vi "HFRR ADV v04.vi"() -> ()   [LabVIEW 2025] (continued)
              n1369 = String Subset(string=w1178, offset (0)=45, length (rest)=9 ("length (rest)")) -> (substring=w1193:string)
              n1370 = Fract/Exp String To Number(string=w1193) -> (number=w1190:dbl)  [unwired: 3 in, 1 out]
              n1371 = String Subset(string=w1178, offset (0)=55, length (rest)=9 ("length (rest)")) -> (substring=w1187:string)
              n1372 = Fract/Exp String To Number(string=w1187) -> (number=w1186:dbl)  [unwired: 3 in, 1 out]
              n1373 = String Subset(string=w1178, offset (0)=25, length (rest)=9 ("length (rest)")) -> (substring=w1185:string)
              n1374 = Fract/Exp String To Number(string=w1185) -> (number=w1182:dbl)  [unwired: 3 in, 1 out]
              n1375 = String Subset(string=w1178, offset (0)=85, length (rest)=9 ("length (rest)")) -> (substring=w1179:string)
              n1376 = Fract/Exp String To Number(string=w1179) -> (number=w1177:dbl)  [unwired: 3 in, 1 out]
            }
            n1377 = Delete From Array(array=w1017, index=0) -> (array with subset deleted=w900:dbl[])  [unwired: 1 in, 1 out]
            n1378 = Delete From Array(array=w1009, index=0) -> (array with subset deleted=w898:dbl[])  [unwired: 1 in, 1 out]
            n1379 = Delete From Array(array=w1027, index=0) -> (array with subset deleted=w902:dbl[])  [unwired: 1 in, 1 out]
            n1380 = Delete From Array(array=w1007, index=0) -> (array with subset deleted=w987:dbl[])  [unwired: 1 in, 1 out]
            n1381 = Delete From Array(array=w977, index=0) -> (array with subset deleted=w904:dbl[])  [unwired: 1 in, 1 out]
            n1382 = Delete From Array(array=w1015, index=0) -> (array with subset deleted=w988:dbl[])  [unwired: 1 in, 1 out]
            n1383 = Delete From Array(array=w1025, index=0) -> (array with subset deleted=w986:dbl[])  [unwired: 1 in, 1 out]
            n1384 = Delete From Array(array=w1034, index=0) -> (array with subset deleted=w989:dbl[])  [unwired: 1 in, 1 out]
            n1385 = Bundle "Bundle"(w898, w987) -> (w1052:cluster{dbl[], dbl[]})  [unwired: 1 in]
            n1386 = Bundle "Bundle"(w902, w986) -> (w1054:cluster{dbl[], dbl[]})  [unwired: 1 in]
            n1387 = Bundle "Bundle"(w900, w988) -> (w1053:cluster{dbl[], dbl[]})  [unwired: 1 in]
            n1388 = Bundle "Bundle"(w904, w989) -> (w923:cluster{dbl[], dbl[]})  [unwired: 1 in]
            n1389 = Build Array "Build Array"(w923, w1054, w1053, w1052) -> (→"Coefficient Of Friction":cluster{dbl[], dbl[]}[])
            n1390 = Delete From Array(array=w1022, index=0) -> (array with subset deleted=w1023:dbl[])  [unwired: 1 in, 1 out]
            n1391 = Delete From Array(array=w1004, index=0) -> (array with subset deleted=w1005:dbl[])  [unwired: 1 in, 1 out]
            n1392 = Delete From Array(array=w1013, index=0) -> (array with subset deleted=w1014:dbl[])  [unwired: 1 in, 1 out]
            n1393 = Delete From Array(array=w1031, index=0) -> (array with subset deleted=w1032:dbl[])  [unwired: 1 in, 1 out]
            n1394 = Delete From Array(array=w1002, index=0) -> (array with subset deleted=w932:dbl[])  [unwired: 1 in, 1 out]
            n1395 = Delete From Array(array=w1011, index=0) -> (array with subset deleted=w933:dbl[])  [unwired: 1 in, 1 out]
            n1396 = Delete From Array(array=w1029, index=0) -> (array with subset deleted=w935:dbl[])  [unwired: 1 in, 1 out]
            n1397 = Delete From Array(array=w1020, index=0) -> (array with subset deleted=w934:dbl[])  [unwired: 1 in, 1 out]
            n1398 = Bundle "Bundle"(w898, w932) -> (w1044:cluster{dbl[], dbl[]})  [unwired: 1 in]
            n1399 = Bundle "Bundle"(w902, w934) -> (w1045:cluster{dbl[], dbl[]})  [unwired: 1 in]
            n1400 = Bundle "Bundle"(w900, w933) -> (w1043:cluster{dbl[], dbl[]})  [unwired: 1 in]
            n1401 = Bundle "Bundle"(w904, w935) -> (w922:cluster{dbl[], dbl[]})  [unwired: 1 in]
            n1402 = Delete From Array(array=w995, index=0) -> (array with subset deleted=w983:dbl[])  [unwired: 1 in, 1 out]
            n1403 = Build Array "Build Array"(w922, w1045, w1043, w1044) -> (→"Air Temperature":cluster{dbl[], dbl[]}[])
            n1404 = Delete From Array(array=w1000, index=0) -> (array with subset deleted=w985:dbl[])  [unwired: 1 in, 1 out]
            "array w/ subset deleted" <- w985
            n1405 = Delete From Array(array=w998, index=0) -> (array with subset deleted=w984:dbl[])  [unwired: 1 in, 1 out]
            n1406 = Delete From Array(array=w975, index=0) -> (array with subset deleted=w931:dbl[])  [unwired: 1 in, 1 out]
            n1407 = Bundle "Bundle"(w898, w1005) -> (w1037:cluster{dbl[], dbl[]})  [unwired: 1 in]
            n1408 = Bundle "Bundle"(w902, w1023) -> (w1036:cluster{dbl[], dbl[]})  [unwired: 1 in]
            n1409 = Bundle "Bundle"(w900, w1014) -> (w1038:cluster{dbl[], dbl[]})  [unwired: 1 in]
            n1410 = Bundle "Bundle"(w904, w1032) -> (w896:cluster{dbl[], dbl[]})  [unwired: 1 in]
            n1411 = Build Array "Build Array"(w896, w1036, w1038, w1037) -> (→"XY Graph 13":cluster{dbl[], dbl[]}[])
            n1412 = Delete From Array(array=w994, index=0) -> (array with subset deleted=w982:dbl[])  [unwired: 1 in, 1 out]
            n1413 = Delete From Array(array=w969, index=0) -> (array with subset deleted=w928:dbl[])  [unwired: 1 in, 1 out]
            n1414 = Delete From Array(array=w973, index=0) -> (array with subset deleted=w930:dbl[])  [unwired: 1 in, 1 out]
            n1415 = Delete From Array(array=w971, index=0) -> (array with subset deleted=w929:dbl[])  [unwired: 1 in, 1 out]
            n1416 = call-poly <vilib>:"Mean.vi"("X"=w987) -> ("mean"=→"КОФ4":dbl)  [unwired: 1 out]
            n1417 = call-poly <vilib>:"Mean.vi"("X"=w989) -> ("mean"=→"КОФ1":dbl)  [unwired: 1 out]
            n1418 = call-poly <vilib>:"Mean.vi"("X"=w988) -> ("mean"=→"КОФ3":dbl)  [unwired: 1 out]
            n1419 = Bundle "Bundle"(w904, w985) -> (w918:cluster{dbl[], dbl[]})  [unwired: 1 in]
            n1420 = Bundle "Bundle"(w898, w982) -> (w990:cluster{dbl[], dbl[]})  [unwired: 1 in]
            n1421 = Bundle "Bundle"(w902, w984) -> (w992:cluster{dbl[], dbl[]})  [unwired: 1 in]
            n1422 = Bundle "Bundle"(w900, w983) -> (w991:cluster{dbl[], dbl[]})  [unwired: 1 in]
            n1423 = call-poly <vilib>:"Mean.vi"("X"=w986) -> ("mean"=→"КОФ2":dbl)  [unwired: 1 out]
            n1424 = Build Array "Build Array"(w918, w992, w991, w990) -> (→"Sample Temperature":cluster{dbl[], dbl[]}[])
            n1425 = Bundle "Bundle"(w904, w931) -> (w895:cluster{dbl[], dbl[]})  [unwired: 1 in]
            n1426 = Bundle "Bundle"(w898, w928) -> (w966:cluster{dbl[], dbl[]})  [unwired: 1 in]
            n1427 = Bundle "Bundle"(w902, w930) -> (w968:cluster{dbl[], dbl[]})  [unwired: 1 in]
            n1428 = Bundle "Bundle"(w900, w929) -> (w967:cluster{dbl[], dbl[]})  [unwired: 1 in]
            n1429 = Delete From Array(array=w954, index=0) -> (array with subset deleted=w926:dbl[])  [unwired: 1 in, 1 out]
            n1430 = Delete From Array(array=w952, index=0) -> (array with subset deleted=w925:dbl[])  [unwired: 1 in, 1 out]
            n1431 = call-poly <vilib>:"Mean.vi"("X"=w984) -> ("mean"=→"CP2":dbl)  [unwired: 1 out]
            n1432 = call-poly <vilib>:"Mean.vi"("X"=w982) -> ("mean"=→"CP4":dbl)  [unwired: 1 out]
            n1433 = Build Array "Build Array"(w895, w968, w967, w966) -> (→"Humidity":cluster{dbl[], dbl[]}[])
            n1434 = call-poly <vilib>:"Mean.vi"("X"=w983) -> ("mean"=→"CP3":dbl)  [unwired: 1 out]
            n1435 = call-poly <vilib>:"Mean.vi"("X"=w985) -> ("mean"=→"CP1":dbl)  [unwired: 1 out]
            n1436 = Delete From Array(array=w956, index=0) -> (array with subset deleted=w927:dbl[])  [unwired: 1 in, 1 out]
            n1437 = Bundle "Bundle"(w935, w931) -> (w937:cluster{dbl[], dbl[]})  [unwired: 1 in]
            n1438 = Bundle "Bundle"(w932, w928) -> (w940:cluster{dbl[], dbl[]})  [unwired: 1 in]
            n1439 = Bundle "Bundle"(w934, w930) -> (w938:cluster{dbl[], dbl[]})  [unwired: 1 in]
            n1440 = Bundle "Bundle"(w933, w929) -> (w939:cluster{dbl[], dbl[]})  [unwired: 1 in]
            n1441 = Delete From Array(array=w950, index=0) -> (array with subset deleted=w924:dbl[])  [unwired: 1 in, 1 out]
            n1442 = Build Array "Build Array"(w937, w938, w939, w940) -> (→"Air Temp vs Rh":cluster{dbl[], dbl[]}[])
            n1443 = Build Array "Build Array"(w895, w918) -> (w921:cluster{dbl[], dbl[]}[])
            "XY Graph 17" <- w921
            n1444 = local write "XY Graph 16"(w921) -> ()
            n1445 = Bundle "Bundle"(w902, w926) -> (w948:cluster{dbl[], dbl[]})  [unwired: 1 in]
            n1446 = Bundle "Bundle"(w900, w925) -> (w947:cluster{dbl[], dbl[]})  [unwired: 1 in]
            n1447 = Bundle "Bundle"(w898, w924) -> (w946:cluster{dbl[], dbl[]})  [unwired: 1 in]
            n1448 = Bundle "Bundle"(w904, w927) -> (w949:cluster{dbl[], dbl[]})  [unwired: 1 in]
            n1449 = Delete From Array(array=w916, index=0) -> (array with subset deleted=w903:dbl[])  [unwired: 1 in, 1 out]
            n1450 = Delete From Array(array=w912, index=0) -> (array with subset deleted=w901:dbl[])  [unwired: 1 in, 1 out]
            n1451 = Build Array "Build Array"(w949, w948, w947, w946) -> (→"Stroke":cluster{dbl[], dbl[]}[])
            n1452 = Delete From Array(array=w910, index=0) -> (array with subset deleted=w897:dbl[])  [unwired: 1 in, 1 out]
            n1453 = Delete From Array(array=w911, index=0) -> (array with subset deleted=w899:dbl[])  [unwired: 1 in, 1 out]
            n1454 = Bundle "Bundle"(w904, w903) -> (w909:cluster{dbl[], dbl[]})  [unwired: 1 in]
            n1455 = Bundle "Bundle"(w902, w901) -> (w908:cluster{dbl[], dbl[]})  [unwired: 1 in]
            n1456 = call-poly <vilib>:"Mean.vi"("X"=w927) -> ("mean"=→"КОФ2 2":dbl)  [unwired: 1 out]
            n1457 = Bundle "Bundle"(w898, w897) -> (w906:cluster{dbl[], dbl[]})  [unwired: 1 in]
            n1458 = Bundle "Bundle"(w900, w899) -> (w907:cluster{dbl[], dbl[]})  [unwired: 1 in]
            n1459 = call-poly <vilib>:"Mean.vi"("X"=w926) -> ("mean"=→"КОФ2 3":dbl)  [unwired: 1 out]
            n1460 = call-poly <vilib>:"Mean.vi"("X"=w924) -> ("mean"=→"КОФ2 5":dbl)  [unwired: 1 out]
            n1461 = call-poly <vilib>:"Mean.vi"("X"=w925) -> ("mean"=→"КОФ2 4":dbl)  [unwired: 1 out]
            n1462 = Build Array "Build Array"(w909, w908, w907, w906) -> (→"Frequency":cluster{dbl[], dbl[]}[])
          }
          frame #2 {
          }
          frame #3 {
            n1463 = local read "String Control 4"() -> (w1220:string)
            n1464 = local read "String Control 6"() -> (w1219:string)
            n1465 = local read "String Control 8"() -> (w1218:string)
            n1466 = local read "String Control 2"() -> (w1221:string)
            n1467 = property on="OPEN" class="Bool (strict)"("Visible"=TRUE) -> ()  [unwired: 2 in, 2 out]
            n1468 = Match Pattern(string=w1219, regular expression="Frequency :- ") -> (after substring=w1244:string)  [unwired: 1 in, 3 out]
            n1469 = Match Pattern(string=w1221, regular expression="Frequency :- ") -> (after substring=w1254:string)  [unwired: 1 in, 3 out]
            n1470 = Match Pattern(string=w1220, regular expression="Frequency :- ") -> (after substring=w1249:string)  [unwired: 1 in, 3 out]
            n1471 = Match Pattern(string=w1218, regular expression="Frequency :- ") -> (after substring=w1239:string)  [unwired: 1 in, 3 out]
            n1472 = String Subset(string=w1244, length (rest)=9 ("length (rest)")) -> (substring=w1246:string)  [unwired: 1 in]
            n1473 = String Subset(string=w1254, length (rest)=9 ("length (rest)")) -> (substring=w1256:string)  [unwired: 1 in]
            n1474 = String Subset(string=w1249, length (rest)=9 ("length (rest)")) -> (substring=w1251:string)  [unwired: 1 in]
            n1475 = String Subset(string=w1239, length (rest)=9 ("length (rest)")) -> (substring=w1241:string)  [unwired: 1 in]
            n1476 = Fract/Exp String To Number(string=w1246) -> (number=w1247:dbl)  [unwired: 3 in, 1 out]
            n1477 = Fract/Exp String To Number(string=w1256) -> (number=w1257:dbl)  [unwired: 3 in, 1 out]
            n1478 = Fract/Exp String To Number(string=w1251) -> (number=w1252:dbl)  [unwired: 3 in, 1 out]
            n1479 = Fract/Exp String To Number(string=w1241) -> (number=w1242:dbl)  [unwired: 3 in, 1 out]
            n1480 = local write "freq3"(w1247) -> ()
            n1481 = local write "freq2"(w1252) -> ()
            n1482 = local write "freq1"(w1257) -> ()
            n1483 = local write "freq 4"(w1242) -> ()
            n1484 = local write "Numeric 13"(0 ("Numeric 13")) -> ()
            n1485 = local write "Numeric 11"(0 ("Numeric 11")) -> ()
            n1486 = local write "Numeric 8"(0 ("Numeric 8")) -> ()
            n1487 = local write "Numeric 12"(0 ("Numeric 12")) -> ()
            n1488 = Match Pattern(string=w1219, regular expression="Samples / cycle :- ") -> (after substring=w1227:string)  [unwired: 1 in, 3 out]
            n1489 = Match Pattern(string=w1221, regular expression="Samples / cycle :- ") -> (after substring=w1235:string)  [unwired: 1 in, 3 out]
            n1490 = Match Pattern(string=w1220, regular expression="Samples / cycle :- ") -> (after substring=w1231:string)  [unwired: 1 in, 3 out]
            n1491 = Match Pattern(string=w1218, regular expression="Samples / cycle :- ") -> (after substring=w1223:string)  [unwired: 1 in, 3 out]
            n1492 = String Subset(string=w1227, length (rest)=6 ("length (rest)")) -> (substring=w1229:string)  [unwired: 1 in]
            n1493 = String Subset(string=w1235, length (rest)=6 ("length (rest)")) -> (substring=w1237:string)  [unwired: 1 in]
            n1494 = String Subset(string=w1231, length (rest)=6 ("length (rest)")) -> (substring=w1233:string)  [unwired: 1 in]
            n1495 = String Subset(string=w1223, length (rest)=6 ("length (rest)")) -> (substring=w1225:string)  [unwired: 1 in]
            n1496 = Fract/Exp String To Number(string=w1229) -> (number=w1215:dbl)  [unwired: 3 in, 1 out]
            n1497 = Fract/Exp String To Number(string=w1237) -> (number=w1217:dbl)  [unwired: 3 in, 1 out]
            n1498 = Fract/Exp String To Number(string=w1233) -> (number=w1216:dbl)  [unwired: 3 in, 1 out]
            n1499 = Fract/Exp String To Number(string=w1225) -> (number=w1214:dbl)  [unwired: 3 in, 1 out]
            n1500 = local write "sample2"(w1216) -> ()
            n1501 = local write "sample3"(w1215) -> ()
            n1502 = local write "sample1"(w1217) -> ()
            n1503 = local write "sample4"(w1214) -> ()
          }
        }
      }
    }
    n1504 = Wait (ms)(milliseconds to wait=u32 50) -> ()  [unwired: 1 out]
    n1505 = property on="STOP 3" class="Bool (strict)"() -> ("Visible"=w828:bool)  [unwired: 2 in, 2 out]
    n1506 = case shown="True" w828 {
      frame False {
      }
      frame True {
        n1507 = case shown="True" "Save Results" {
          frame False {
          }
          frame True {
            w1738 = "\r"
            n1508 = local read "Temperature before test"() -> (w1776:dbl)
            n1509 = local read "Temperature after test"() -> (w1778:dbl)
            n1510 = local read "Humidity before test"() -> (w1775:dbl)
            n1511 = local read "Humidity after test"() -> (w1777:dbl)
            n1512 = local read "MWSD"() -> (w1779:dbl)
            n1513 = local read "WS1.4"() -> (w1782:dbl)
            n1514 = local read "AVP"() -> (w1780:dbl)
            n1515 = local read "HCF"() -> (w1781:dbl)
            n1516 = local write "Save Results"(FALSE ("OK Button 5")) -> ()
            n1517 = Number To Fractional String(number=w1778, width (-)=i16 6, precision (6)=i16 1) -> (F-format string=w1756:string)  [unwired: 1 in]
            n1518 = Number To Fractional String(number=w1779, width (-)=i16 6, precision (6)=i16 1) -> (F-format string=w1753:string)  [unwired: 1 in]
            n1519 = Number To Fractional String(number=w1780, width (-)=i16 6, precision (6)=i16 3) -> (F-format string=w1749:string)  [unwired: 1 in]
            n1520 = Number To Fractional String(number=w1777, width (-)=i16 6, precision (6)=i16 1) -> (F-format string=w1760:string)  [unwired: 1 in]
            n1521 = Number To Fractional String(number=w1781, width (-)=i16 6, precision (6)=i16 2) -> (F-format string=w1747:string)  [unwired: 1 in]
            n1522 = Number To Fractional String(number=w1782, width (-)=i16 6, precision (6)=i16 1) -> (F-format string=w1742:string)  [unwired: 1 in]
            n1523 = Number To Fractional String(number=w1776, width (-)=i16 6, precision (6)=i16 1) -> (F-format string=w1764:string)  [unwired: 1 in]
            n1524 = Number To Fractional String(number=w1775, width (-)=i16 6, precision (6)=i16 1) -> (F-format string=w1767:string)  [unwired: 1 in]
            n1525 = local read "String"() -> (w1771:string)
            n1526 = local read "FILE"() -> (w1774:string)
            n1527 = Concatenate Strings(w1771, w1774) -> (w1793:string)
            n1528 = Concatenate Strings(w1793, ".dwm" ("Substring")) -> (w1791:string)
            n1529 = Concatenate Strings(w1747, ")" ("string")) -> (w1745:string)
            n1530 = Concatenate Strings("(" ("string"), w1742, ")Microns" ("string")) -> (w1741:string)
            n1531 = Concatenate Strings("(" ("string"), w1767, " ) % RH," ("string")) -> (w1768:string)
            n1532 = Concatenate Strings("(" ("string"), w1749, ")  kPa," ("string")) -> (w1739:string)
            n1533 = String To Path(string=w1791) -> (path=w1790:path)
            n1534 = Concatenate Strings("(" ("string"), w1764, ")  Deg C ," ("string")) -> (w1763:string)
            n1535 = Concatenate Strings("(" ("string"), w1760, " ) % RH," ("string")) -> (w1759:string)
            n1536 = Concatenate Strings("(" ("string"), w1756, ")  Deg C ," ("string")) -> (w1755:string)
            n1537 = Concatenate Strings("(" ("string"), w1753, ")  Microns," ("string")) -> (w1752:string)
            n1538 = local read "REMARKS"() -> (w1773:string)
            "REMARKS 2" <- w1773
            n1539 = Concatenate Strings(w1773, w1738, " Humidity before test= " ("Substring"), w1768, w1738, " Temperature before test = " ("Substring"), w1763, w1738, " Humidity after test= " ("Substring"), w1759, w1738, "Temperature after test = " ("Substring"), w1755, w1738, "MSD = " ("Substring"), w1752, w1738, "  AVP = " ("Substring"), w1739, w1738, "  HCF                     =( " ("Substring"), w1745, w1738, " WS1.4                  = " ("Substring"), w1741, w1738) -> (w1737:string)
            "data" <- w1737
            n1540 = call <vilib>:"Write Characters To File.vi"("append to file? (new file:F)"=FALSE, "character string"=w1737, "file path (dialog if empty)"=w1790) -> ()  [unwired: 2 in, 1 out]
            n1541 = Match Pattern(string=w1737, regular expression="!") -> (after substring=→"export":string)  [unwired: 1 in, 3 out]
          }
        }
        n1542 = local read "Temperature before test"() -> (w1706:dbl)
        n1543 = local read "Humidity before test"() -> (w1708:dbl)
        n1544 = local read "Temperature after test"() -> (w1722:dbl)
        n1545 = Add(x=231.864, y=w1706) -> (x+y=w1703:dbl)
        n1546 = Add(x=231.864, y=w1722) -> (x+y=w1719:dbl)
        n1547 = local read "Humidity after test"() -> (w1724:dbl)
        n1548 = Divide(x=1705.984, y=w1703) -> (x/y=w1704:dbl)
        n1549 = Divide(x=1705.984, y=w1719) -> (x/y=w1720:dbl)
        n1550 = Subtract(x=8.017352 ("y"), y=w1704) -> (x-y=w1733:dbl)
        n1551 = expression code="10**y"(w1733) -> (w1710:dbl)
        n1552 = Subtract(x=8.017352 ("y"), y=w1720) -> (x-y=w1727:dbl)
        n1553 = expression code="10**y"(w1727) -> (w1726:dbl)
        n1554 = Multiply(x=w1708, y=w1710) -> (x*y=w1709:dbl)
        n1555 = Multiply(x=w1724, y=w1726) -> (x*y=w1725:dbl)
        n1556 = Divide(x=w1709, y=750.0) -> (x/y=w1728:dbl)
        n1557 = Divide(x=w1725, y=750.0) -> (x/y=w1729:dbl)
        n1558 = Add(x=w1728, y=w1729) -> (x+y=w1730:dbl)
        n1559 = Divide(x=w1730, y=2.0) -> (x/y=w1732:dbl)
        n1560 = local write "AVP"(w1732) -> ()
        n1561 = local read "HCF"() -> (w1715:dbl)
        n1562 = Subtract(x=1.4, y=w1732) -> (x-y=w1713:dbl)
        n1563 = local read "MWSD"() -> (w1711:dbl)
        n1564 = Multiply(x=w1713, y=w1715) -> (x*y=w1714:dbl)
        n1565 = Add(x=w1714, y=w1711) -> (x+y=→"WS1.4":dbl)
      }
    }
    n1566 = case shown="True" "Prog Uno" {
      frame False {
      }
      frame True {
        n1567 = stacked-sequence {
          frame #0 {
            n1568 = Delete(path (use dialog)=path "C:/LAB-IQ-NXT/UNOCOMPILE.bat" ("working directory")) -> ()  [unwired: 4 in, 3 out]
          }
          frame #1 {
            n1569 = local read "Com Port 1"() -> (w1306:refnum<visa-resource-name>)
            n1570 = Concatenate Strings("cmd.exe /c \"mode " ("command line"), w1306, ":1200,n,8,1\"\n" ("command line")) -> (w1311:string)
            n1571 = Concatenate Strings(w1311, "CD\\\nCD WinDucom\navrdude -C avrdude.conf -v -patmega328p -carduino -P" ("command line"), w1306, " -b115200 -D -Uflash:w:UNO_V20.hex:i\n" ("command line"), "\r") -> (w1313:string)
            "STR" <- w1313
            n1572 = call <vilib>:"Write Characters To File.vi"("append to file? (new file:F)"=FALSE, "character string"=w1313, "file path (dialog if empty)"=path "C:/LAB-IQ-NXT/UNOCOMPILE.bat" ("working directory")) -> ()  [unwired: 2 in, 1 out]
          }
          frame #2 {
            n1573 = disable-structure shown="Disabled" {
              frame Disabled {
                w1317 = "cmd.exe  /c \"C:\\LAB-IQ-NXT\\UNOCOMPILE.bat\"" ("string")
                n1574 = call <vilib>:"System Exec.vi"("expected output size  (4096)"=u32 65535, "run minimized? (F)"=FALSE, "wait until completion? (T)"=TRUE ("run minimized? (F)"), "working directory"=path "C:/LAB-IQ-NXT", "standard input"=w1317, "command line"=w1317) -> ("error out"=w1316:errorcluster, "standard output"=→"String 42":string)  [unwired: 2 in, 2 out]
                "error out 3" <- w1316
                n1575 = local write "Prog Uno"(FALSE ("run minimized? (F)")) -> ()
                n1576 = flat-sequence {
                  tunnel: w1316 -> [_]
                  frame #0 {
                  }
                }
              }
              frame Enabled {
              }
            }
          }
        }
      }
    }
    n1577 = case shown="True" "Prog Due" {
      frame False {
      }
      frame True {
        n1578 = stacked-sequence {
          frame #0 {
            n1579 = Delete(path (use dialog)=path "C:/LAB-IQ-NXT/DUECOMPILE.bat" ("working directory")) -> ()  [unwired: 4 in, 3 out]
          }
          frame #1 {
            n1580 = disable-structure shown="Disabled" {
              frame Disabled {
                n1581 = local read "visa due"() -> (w1288:string)
                n1582 = Concatenate Strings("cmd.exe /c \"mode " ("command line"), w1288, ":1200,n,8,1\"\n" ("command line")) -> (w1293:string)
                n1583 = Concatenate Strings(w1293, "CD\\\nCD WinDucom\nTIMEOUT 1\n bossac.exe -i -d --port=" ("command line"), w1288, " -U false -e -w -v -b DUE.bin -R\n" ("command line"), "\r") -> (w1295:string)
                "concatenated string 2" <- w1295
                n1584 = call <vilib>:"Write Characters To File.vi"("append to file? (new file:F)"=FALSE, "character string"=w1295, "file path (dialog if empty)"=path "C:/LAB-IQ-NXT/DUECOMPILE.bat" ("working directory")) -> ()  [unwired: 2 in, 1 out]
              }
              frame Enabled {
              }
            }
          }
          frame #2 {
            # "C:\\LAB-IQ-NXT\\DUECOMPILE.bat"
            n1585 = disable-structure shown="Disabled" {
              frame Disabled {
                w1300 = "cmd.exe  /c \"C:\\LAB-IQ-NXT\\DUECOMPILE.bat\"" ("string")
                n1586 = call <vilib>:"System Exec.vi"("expected output size  (4096)"=u32 65535, "run minimized? (F)"=FALSE, "wait until completion? (T)"=TRUE ("run minimized? (F)"), "working directory"=path "C:/LAB-IQ-NXT", "standard input"=w1300, "command line"=w1300) -> ("error out"=w1299:errorcluster, "standard output"=→"String 44":string)  [unwired: 2 in, 2 out]
                "error out 4" <- w1299
                n1587 = flat-sequence {
                  tunnel: w1299 -> [_]
                  frame #0 {
                  }
                }
              }
              frame Enabled {
              }
            }
            n1588 = local write "Prog Due"(FALSE ("Prog Due")) -> ()
          }
        }
      }
    }
    n1589 = flat-sequence {
      frame #0 {
        n1590 = local read "x = y?"() -> (w1328:bool)
        n1591 = And(x="EDIT", y=w1328) -> (x .and. y?=w1326:bool)
        n1592 = case shown="True" "SAVE" {
          frame False {
          }
          frame True {
            n1593 = stacked-sequence {
              seq-local: [w1529 _ _] -> [_ w1683 _]
              frame #0 {
                (unwired) i16 5 ("precision (6)")
                # "[CH1]    - FF\n[CH2]   - TEMPERATURE\n[CH3]    - Humidity\n[CH4]    - AIR TEMP\n[CH5]\\- Visa Uno\n[CH6] \\- Visa Due\n[CH7]  \\- file path\n[CH8]   - Displacement Gain\n[CHA]   - Stroke Gain\n[CHB]   - Stroke PID Gain\n[CHC]   -Language Selection\n[CHD]   -Power +\n[CHE]   -Power_\n[CHF]   -Heater\n[CHG]   -Humidity Wet\n[CHH]   -Humidity Dry\n[CHI]   -Integral Time"
                n1594 = local read "Com Port 1"() -> (w1520:refnum<visa-resource-name>)
                n1595 = local read "AIR TEMPERATURE :"() -> (w1516:dbl)
                n1596 = local read "DISPLACEMENT :"() -> (w1514:dbl)
                n1597 = local read "HUMIDITY:"() -> (w1515:dbl)
                n1598 = local read "Com Port 2"() -> (w1519:refnum<visa-resource-name>)
                n1599 = local read "TEMPERATURE :"() -> (w1517:dbl)
                n1600 = local read "Stroke PID Gains"() -> (w1580:T8)
                n1601 = local read "FRIC. FORCE :"() -> (w1518:dbl)
                n1602 = local read "STROKE GAIN :"() -> (w1513:dbl)
                n1603 = Unbundle By Name(w1580) -> ("Proportional Gain (Kc)"=w1579:dbl, "Integral Time (Ti, min)"=w1521:dbl)
                n1604 = local read "CH-HUMIDITY DRY"() -> (w1532:u16)
                n1605 = Path To String(path="File Path") -> (string=w1602:string)
                n1606 = local read "Language Selection"() -> (w1577:enum16{"English", "Russian"})
                n1607 = local read "CH-POWER +"() -> (w1544:u16)
                n1608 = local read "CH-HUMIDITY WET"() -> (w1535:u16)
                n1609 = Number To Fractional String(number=w1515, width (-)=i16 10 ("precision (6)"), precision (6)=i16 5) -> (F-format string=w1627:string)  [unwired: 1 in]
                n1610 = Concatenate Strings(w1602, "\\" ("string")) -> (w1601:string)
                n1611 = local read "CH-POWER -"() -> (w1541:u16)
                n1612 = Number To Fractional String(number=w1517, width (-)=i16 10 ("precision (6)"), precision (6)=i16 5) -> (F-format string=w1633:string)  [unwired: 1 in]
                n1613 = Number To Fractional String(number=w1516, width (-)=i16 10 ("precision (6)"), precision (6)=i16 5) -> (F-format string=w1621:string)  [unwired: 1 in]
                n1614 = Number To Fractional String(number=w1514, width (-)=i16 10 ("precision (6)"), precision (6)=i16 5) -> (F-format string=w1594:string)  [unwired: 1 in]
                n1615 = local read "CH-HEATER"() -> (w1538:u16)
                n1616 = Number To Fractional String(number=w1513, width (-)=i16 10 ("precision (6)"), precision (6)=i16 5) -> (F-format string=w1593:string)  [unwired: 1 in]
                n1617 = Number To Fractional String(number=w1518, width (-)=i16 10 ("precision (6)"), precision (6)=i16 5) -> (F-format string=w1634:string)  [unwired: 1 in]
                n1618 = Number To Fractional String(number=w1579, width (-)=i16 10 ("precision (6)"), precision (6)=i16 5) -> (F-format string=w1581:string)  [unwired: 1 in]
                n1619 = Number To Fractional String(number=w1577, width (-)=i16 10 ("precision (6)"), precision (6)=i16 5) -> (F-format string=w1573:string)  [unwired: 1 in]
                n1620 = Number To Fractional String(number=w1544, width (-)=i16 10 ("precision (6)"), precision (6)=i16 5) -> (F-format string=w1567:string)  [unwired: 1 in]
                n1621 = Number To Fractional String(number=w1541, width (-)=i16 10 ("precision (6)"), precision (6)=i16 5) -> (F-format string=w1564:string)  [unwired: 1 in]
                n1622 = Number To Fractional String(number=w1538, width (-)=i16 10 ("precision (6)"), precision (6)=i16 5) -> (F-format string=w1559:string)  [unwired: 1 in]
                n1623 = Number To Fractional String(number=w1535, width (-)=i16 10 ("precision (6)"), precision (6)=i16 5) -> (F-format string=w1556:string)  [unwired: 1 in]
                n1624 = Number To Fractional String(number=w1532, width (-)=i16 10 ("precision (6)"), precision (6)=i16 5) -> (F-format string=w1551:string)  [unwired: 1 in]
                n1625 = Concatenate Strings("[CH1]" ("string"), w1634, " - FF" ("string"), "\r") -> (w1632:string)
                n1626 = Concatenate Strings("[CH3]" ("string"), w1627, " - Humidity" ("string"), "\r") -> (w1624:string)
                n1627 = Concatenate Strings("[CH7]" ("string"), w1601, "- file path" ("string"), "\r") -> (w1604:string)
                n1628 = Number To Fractional String(number=w1521, width (-)=i16 10 ("precision (6)"), precision (6)=i16 5) -> (F-format string=w1525:string)  [unwired: 1 in]
                n1629 = Concatenate Strings("[CH6]" ("string"), w1519, "- Visa Due" ("string"), "\r") -> (w1605:string)
                n1630 = Concatenate Strings("[CH8]" ("string"), w1594, "- Displacement Gain" ("string"), "\r") -> (w1597:string)
                n1631 = Concatenate Strings("[CHA]" ("string"), w1593, "- Stroke Gain" ("string"), "\r") -> (w1587:string)
                n1632 = Concatenate Strings("[CH5]" ("string"), w1520, "- Visa Uno" ("string"), "\r") -> (w1610:string)
                n1633 = Concatenate Strings("[CH4]" ("string"), w1621, " - AIR TEMP" ("string"), "\r") -> (w1617:string)
                n1634 = Concatenate Strings("[CH2]" ("string"), w1633, " - TEMPERATURE" ("string"), "\r") -> (w1631:string)
                n1635 = Concatenate Strings("[CHC]" ("string"), w1573, "-Language Selection" ("string"), "\r") -> (w1570:string)
                n1636 = Concatenate Strings("[CHD]" ("string"), w1567, "-Power +" ("string"), "\r") -> (w1549:string)
                n1637 = Concatenate Strings("[CHE]" ("string"), w1564, "-Power_" ("string"), "\r") -> (w1548:string)
                n1638 = Concatenate Strings("[CHF]" ("string"), w1559, "-Heater" ("string"), "\r") -> (w1547:string)
                n1639 = Concatenate Strings("[CHB]" ("string"), w1581, "- Stroke PID Gain" ("string"), "\r") -> (w1578:string)
                n1640 = Concatenate Strings("[CHG]" ("string"), w1556, "-Humidity Wet" ("string"), "\r") -> (w1546:string)
                n1641 = Concatenate Strings("[CHH]" ("string"), w1551, "-Humidity Dry" ("string"), "\r") -> (w1545:string)
                n1642 = Concatenate Strings("[CHI]" ("string"), w1525, "-Integral Time " ("string"), "\r") -> (w1522:string)
                n1643 = Concatenate Strings(w1632, w1631, w1624, w1617, w1610, w1605, w1604, w1597, w1587, w1578, w1570, w1549, w1548, w1547, w1546, w1545, w1522) -> (w1529:string)
                "gain" <- w1529
              }
              frame #1 {
                n1644 = local read "AIR TEMP INTERCEPT:"() -> (w1646:dbl)
                n1645 = local read "TEMP INTERCEPT:"() -> (w1645:dbl)
                n1646 = local read "Com Port 3"() -> (w1655:refnum<visa-resource-name>)
                n1647 = local read "LvdtOff"() -> (w1648:dbl)
                n1648 = Number To Fractional String(number=w1645, width (-)=i16 10 ("precision (6)"), precision (6)=i16 5) -> (F-format string=w1671:string)  [unwired: 1 in]
                n1649 = Number To Fractional String(number=w1646, width (-)=i16 10 ("precision (6)"), precision (6)=i16 5) -> (F-format string=w1678:string)  [unwired: 1 in]
                n1650 = Number To Fractional String(number=w1648, width (-)=i16 10 ("precision (6)"), precision (6)=i16 5) -> (F-format string=w1652:string)  [unwired: 1 in]
                n1651 = Concatenate Strings("[CHK]" ("string"), w1671, "-TEMP INTERCEPT" ("string"), "\r") -> (w1667:string)
                n1652 = Concatenate Strings("[CHJ]" ("string"), w1678, "-AIR TEMP INTERCEPT" ("string"), "\r") -> (w1668:string)
                n1653 = Concatenate Strings("[SNO]" ("string"), "S.NO", "-" ("string"), "\r") -> (w1663:string)
                n1654 = Concatenate Strings("[CHL]" ("string"), w1655, "- Visa humid" ("string"), "\r") -> (w1658:string)
                n1655 = Concatenate Strings("[CHI]" ("string"), w1652, "-LVDT Position Offset" ("string"), "\r") -> (w1647:string)
                n1656 = Concatenate Strings(w1683, w1668, w1667, w1663, w1658, w1647) -> (w1682:string)
                n1657 = String To Path(string="C:\\LAB-IQ-NXT\\calibrate WO 2464.dcf") -> (path=w1656:path)
                n1658 = call <vilib>:"Write Characters To File.vi"("append to file? (new file:F)"=FALSE, "character string"=w1682, "file path (dialog if empty)"=w1656) -> ()  [unwired: 2 in, 1 out]
              }
              frame #2 {
                n1659 = local write "Lan flag"(0.0 ("Lan flag")) -> ()
                n1660 = local write "Re-Initialise"(TRUE ("Re-Initialise")) -> ()
                n1661 = local write "conststatus"(0.0 ("rpm value : 2")) -> ()
                n1662 = local write "SAVE"(FALSE ("OK Button 14")) -> ()
              }
            }
          }
        }
        n1663 = case shown="False" w1326 {
          tunnel: [u8 2 ("Disabled") u8 0 ("Disabled")] -> w1325
          tunnel: [w1688 TRUE ("Visible")] -> w1324
          frame False {
            w1688 = FALSE ("Visible")
            n1664 = local write "EDIT 2"(w1688) -> ()
          }
          frame True {
          }
        }
        n1665 = property on="Tab Control" class="TabCtl (strict)"("Visible"=w1324) -> ()  [unwired: 2 in, 2 out]
        n1666 = property on="EDIT 2" class="Bool (strict)"("Visible"=w1324) -> ()  [unwired: 2 in, 2 out]
        n1667 = property on="TEMPERATURE :" class="DigNum (strict)"("Disabled"=w1325) -> ()  [unwired: 2 in, 2 out]
        n1668 = property on="SAVE" class="Bool (strict)"("Visible"=w1324) -> ()  [unwired: 2 in, 2 out]
        n1669 = property on="AIR TEMPERATURE :" class="DigNum (strict)"("Disabled"=w1325) -> ()  [unwired: 2 in, 2 out]
        n1670 = property on="SPEED OUT:" class="DigNum (strict)"("Disabled"=w1325) -> ()  [unwired: 2 in, 2 out]
        n1671 = property on="HUMIDITY:" class="DigNum (strict)"("Disabled"=w1325) -> ()  [unwired: 2 in, 2 out]
        n1672 = property on="FRIC. FORCE :" class="DigNum (strict)"("Disabled"=w1325) -> ()  [unwired: 2 in, 2 out]
        n1673 = property on="Tab Control 7" class="TabCtl (strict)"("Disabled"=w1325) -> ()  [unwired: 2 in, 2 out]
        n1674 = property on="Language Selection" class="Enum (strict)"("Visible"=w1324) -> ()  [unwired: 2 in, 2 out]
        n1675 = property on="File Path" class="Path"("Disabled"=w1325) -> ()  [unwired: 2 in, 2 out]
        n1676 = property on="TEMP INTERCEPT:" class="DigNum (strict)"("Disabled"=w1325) -> ()  [unwired: 2 in, 2 out]
        n1677 = property on="visa due" class="CmbBox"("Disabled"=w1325) -> ()  [unwired: 2 in, 2 out]
        n1678 = property on="AIR TEMP INTERCEPT:" class="DigNum (strict)"("Disabled"=w1325) -> ()  [unwired: 2 in, 2 out]
        n1679 = property on="CH-HUMIDITY DRY" class="DigNum (strict)"("Disabled"=w1325) -> ()  [unwired: 2 in, 2 out]
        n1680 = property on="CH-HUMIDITY WET" class="DigNum (strict)"("Disabled"=w1325) -> ()  [unwired: 2 in, 2 out]
        n1681 = property on="CH-POWER -" class="DigNum (strict)"("Disabled"=w1325) -> ()  [unwired: 2 in, 2 out]
        n1682 = property on="CH-HEATER" class="DigNum (strict)"("Disabled"=w1325) -> ()  [unwired: 2 in, 2 out]
        n1683 = property on="CH-POWER +" class="DigNum (strict)"("Disabled"=w1325) -> ()  [unwired: 2 in, 2 out]
        n1684 = property on="SrvM CP" class="Bool (strict)"("Disabled"=w1325) -> ()  [unwired: 2 in, 2 out]
        n1685 = property on="Stroke PID Gains" class="Clust (strict)"("Disabled"=w1325) -> ()  [unwired: 2 in, 2 out]
        n1686 = property on="STROKE GAIN :" class="DigNum (strict)"("Disabled"=w1325) -> ()  [unwired: 2 in, 2 out]
        n1687 = property on="LvdtOff" class="DigNum (strict)"("Disabled"=w1325) -> ()  [unwired: 2 in, 2 out]
        n1688 = property on="DISPLACEMENT :" class="DigNum (strict)"("Disabled"=w1325) -> ()  [unwired: 2 in, 2 out]
        n1689 = property on="Port 2 Error" class="Clust (strict)"("Visible"="EDIT") -> ()  [unwired: 2 in, 2 out]
        n1690 = property on="Port 1 Error" class="Clust (strict)"("Visible"="EDIT") -> ()  [unwired: 2 in, 2 out]
        n1691 = stacked-sequence {
          frame #0 {
            n1692 = local read "EDIT"() -> (w1376:bool)
            n1693 = case shown="True" w1376 {
              tunnel: [u8 2 ("Disabled") u8 0 ("Disabled")] -> _
              frame False {
                w1378 = FALSE
                n1694 = local write "Password"("") -> ()
                n1695 = property on="ENTER THE NEW PASSWORD" class="Str"("Visible"=w1378) -> ()  [unwired: 2 in, 2 out]
                n1696 = property on="ENTER CURRENT PASSWORD" class="Str"("Visible"=w1378) -> ()  [unwired: 2 in, 2 out]
                n1697 = property on="SrvM CP" class="Bool (strict)"("Visible"=w1378) -> ()  [unwired: 2 in, 2 out]
                n1698 = property on="Password" class="Str"("Visible"=w1378) -> ()  [unwired: 2 in, 2 out]
                n1699 = local write "x = y?"(w1378) -> ()
                n1700 = local write "SrvM CP"(w1378) -> ()
                n1701 = property on="message" class="Str"("Visible"=w1378) -> ()  [unwired: 2 in, 2 out]
              }
              frame True {
                w1381 = TRUE
                n1702 = property on="SrvM CP" class="Bool (strict)"("Visible"=w1381) -> ()  [unwired: 2 in, 2 out]
                n1703 = property on="Password" class="Str"("Visible"=w1381) -> ()  [unwired: 2 in, 2 out]
              }
            }
            "dipl pwd" <- "@143$\n" ("dipl pwd")
          }
          frame #1 {
            # "Gain password"
            n1704 = String To Byte Array(string="ENTER CURRENT PASSWORD") -> (unsigned byte array=w1386:u8[])
            n1705 = Search 1D Array(1D array=w1386, element=u8 10) -> (index of element=w1389:i32)  [unwired: 1 in]
            n1706 = Index Array(array=w1386, index=w1389) -> (element=w1385:u8)
            n1707 = Equal?(x=w1385, y=10) -> (x = y?=w1383:bool)
            n1708 = case shown="True" w1383 {
              frame False {
                n1709 = property on="ENTER THE NEW PASSWORD" class="Str"("Visible"=FALSE) -> ()  [unwired: 2 in, 2 out]
              }
              frame True {
                # "password"
                # "change password logic"
                n1710 = local read "dipl pwd"() -> (w1396:string)
                n1711 = local read "ENTER CURRENT PASSWORD"() -> (w1402:string)
                n1712 = String To Byte Array(string=w1402) -> (unsigned byte array=w1404:u8[])
                n1713 = Array Size(array=w1404) -> (size(s)=w1401:i32)
                n1714 = String To Byte Array(string=w1396) -> (unsigned byte array=w1397:u8[])
                n1715 = Array Size(array=w1397) -> (size(s)=w1399:i32)
                n1716 = for {
                  N: w1401 -> [_]
                  tunnel: w1404 -> [w1428]
                  tunnel: [w1426] -> w1405 mode=indexing
                  tunnel: w1401 -> [w1420]
                  i -> [w1421]
                  n1717 = Decrement(x=w1420) -> (x-1=w1418:i32)
                  n1718 = Index Array(array=w1428, index=w1421) -> (element=w1422:u8)
                  n1719 = Equal?(x=w1421, y=w1418) -> (x = y?=w1419:bool)
                  n1720 = Number To Decimal String(number=w1422) -> (decimal integer string=w1427:string)  [unwired: 1 in]
                  n1721 = Select(t="", s=w1419, f="\r") -> (s? t:f=w1424:string)
                  n1722 = Concatenate Strings(w1427, w1424) -> (w1426:string)
                }
                n1723 = for {
                  N: w1399 -> [_]
                  tunnel: w1397 -> [w1416]
                  tunnel: [w1414] -> w1398 mode=indexing
                  tunnel: w1399 -> [w1411]
                  i -> [w1412]
                  n1724 = Decrement(x=w1411) -> (x-1=w1410:i32)
                  n1725 = Index Array(array=w1416, index=w1412) -> (element=w1415:u8)
                  n1726 = Equal?(x=w1412, y=w1410) -> (x = y?=w1409:bool)
                  n1727 = Number To Decimal String(number=w1415) -> (decimal integer string=w1413:string)  [unwired: 1 in]
                  n1728 = Select(t="", s=w1409, f="\r") -> (s? t:f=w1406:string)
                  n1729 = Concatenate Strings(w1413, w1406) -> (w1414:string)
                }
                n1730 = local read "string"() -> (w1403:string)
                n1731 = Concatenate Strings(w1405) -> (w1393:string)
                n1732 = Concatenate Strings(w1398) -> (w1392:string)
                n1733 = Concatenate Strings(w1403) -> (w1400:string)
                n1734 = Equal?(x=w1393, y=w1392) -> (x = y?=w1391:bool)
                n1735 = Equal?(x=w1393, y=w1400) -> (x = y?=w1395:bool)
                n1736 = Or(x=w1395, y=w1391) -> (x .or. y?=w1394:bool)
                n1737 = case shown="True" w1394 {
                  frame False {
                  }
                  frame True {
                    n1738 = property on="ENTER THE NEW PASSWORD" class="Str"("Visible"=TRUE) -> ()  [unwired: 2 in, 2 out]
                  }
                }
              }
            }
          }
          frame #2 {
            n1739 = String To Byte Array(string="ENTER THE NEW PASSWORD") -> (unsigned byte array=w1431:u8[])
            n1740 = Search 1D Array(1D array=w1431, element=u8 10) -> (index of element=w1435:i32)  [unwired: 1 in]
            n1741 = Index Array(array=w1431, index=w1435) -> (element=w1433:u8)
            n1742 = Equal?(x=w1433, y=10) -> (x = y?=w1430:bool)
            n1743 = case shown="True" w1430 {
              frame False {
              }
              frame True {
                n1744 = local read "ENTER THE NEW PASSWORD"() -> (w1438:string)
                n1745 = String To Byte Array(string=w1438) -> (unsigned byte array=w1443:u8[])
                n1746 = Array Size(array=w1443) -> (size(s)=w1440:i32)
                n1747 = for {
                  N: w1440 -> [_]
                  tunnel: w1443 -> [w1456]
                  tunnel: [w1453] -> w1445 mode=indexing
                  tunnel: w1440 -> [w1448]
                  i -> [w1446]
                  n1748 = Index Array(array=w1456, index=w1446) -> (element=w1455:u8)
                  n1749 = Decrement(x=w1448) -> (x-1=w1449:i32)
                  n1750 = Equal?(x=w1446, y=w1449) -> (x = y?=w1450:bool)
                  n1751 = Number To Decimal String(number=w1455) -> (decimal integer string=w1454:string)  [unwired: 1 in]
                  n1752 = Select(t="", s=w1450, f="\r") -> (s? t:f=w1447:string)
                  n1753 = Concatenate Strings(w1454, w1447) -> (w1453:string)
                }
                n1754 = local write "SrvM CP"(FALSE) -> ()
                n1755 = local write "EDIT"(FALSE) -> ()
                n1756 = local read "file path"() -> (w1437:path)
                n1757 = Concatenate Strings(w1445) -> (w1439:string)
                n1758 = Delete(path (use dialog)=w1437) -> (deleted path=w1441:path)  [unwired: 4 in, 2 out]
                n1759 = call <vilib>:"Write Characters To File.vi"("append to file? (new file:F)"=FALSE, "character string"=w1439, "file path (dialog if empty)"=w1441) -> ()  [unwired: 2 in, 1 out]
              }
            }
          }
          frame #3 {
            n1760 = case shown="True" "SrvM CP" {
              frame False {
                w1459 = ""
                n1761 = property on="ENTER CURRENT PASSWORD" class="Str"("Visible"=FALSE) -> ()  [unwired: 2 in, 2 out]
                n1762 = local write "ENTER CURRENT PASSWORD"(w1459) -> ()
                n1763 = local write "ENTER THE NEW PASSWORD"(w1459) -> ()
              }
              frame True {
                n1764 = property on="ENTER THE NEW PASSWORD" class="Str"() -> ("Visible"=w1460:bool)  [unwired: 2 in, 2 out]
                n1765 = Not(x=w1460) -> (.not. x?=w1461:bool)
                n1766 = property on="ENTER CURRENT PASSWORD" class="Str"("Visible"=w1461) -> ()  [unwired: 2 in, 2 out]
              }
            }
          }
          frame #4 {
            n1767 = String To Byte Array(string="Password") -> (unsigned byte array=w1468:u8[])
            n1768 = Search 1D Array(1D array=w1468, element=u8 10) -> (index of element=w1466:i32)  [unwired: 1 in]
            n1769 = Index Array(array=w1468, index=w1466) -> (element=w1467:u8)
            n1770 = Equal?(x=w1467, y=10) -> (x = y?=w1463:bool)
            n1771 = case shown="False" w1463 {
              frame False {
              }
              frame True {
                # "password"
                # "password"
                n1772 = local read "Password"() -> (w1481:string)
                n1773 = String To Byte Array(string=w1481) -> (unsigned byte array=w1484:u8[])
                n1774 = Array Size(array=w1484) -> (size(s)=w1479:i32)
                n1775 = local read "file path"() -> (w1469:path)
                n1776 = for {
                  N: w1479 -> [_]
                  tunnel: w1484 -> [w1501]
                  tunnel: [w1499] -> w1485 mode=indexing
                  tunnel: w1479 -> [w1496]
                  i -> [w1497]
                  n1777 = Decrement(x=w1496) -> (x-1=w1495:i32)
                  n1778 = Index Array(array=w1501, index=w1497) -> (element=w1500:u8)
                  n1779 = Equal?(x=w1497, y=w1495) -> (x = y?=w1494:bool)
                  n1780 = Number To Decimal String(number=w1500) -> (decimal integer string=w1498:string)  [unwired: 1 in]
                  n1781 = Select(t="", s=w1494, f="\r") -> (s? t:f=w1491:string)
                  n1782 = Concatenate Strings(w1498, w1491) -> (w1499:string)
                }
                n1783 = String To Byte Array(string="@143$\n") -> (unsigned byte array=w1470:u8[])
                n1784 = Array Size(array=w1470) -> (size(s)=w1475:i32)
                n1785 = call <vilib>:"Read Characters From File.vi"("file path (dialog if empty)"=w1469) -> ("character string"=w1483:string)  [unwired: 5 in, 3 out]
                "string" <- w1483
                n1786 = for {
                  N: w1475 -> [_]
                  tunnel: w1470 -> [w1512]
                  tunnel: [w1510] -> w1473 mode=indexing
                  tunnel: w1475 -> [w1507]
                  i -> [w1508]
                  n1787 = Decrement(x=w1507) -> (x-1=w1506:i32)
                  n1788 = Index Array(array=w1512, index=w1508) -> (element=w1511:u8)
                  n1789 = Equal?(x=w1508, y=w1506) -> (x = y?=w1505:bool)
                  n1790 = Number To Decimal String(number=w1511) -> (decimal integer string=w1509:string)  [unwired: 1 in]
                  n1791 = Select(t="", s=w1505, f="\r") -> (s? t:f=w1502:string)
                  n1792 = Concatenate Strings(w1509, w1502) -> (w1510:string)
                }
                n1793 = Concatenate Strings(w1485) -> (w1477:string)
                n1794 = Concatenate Strings(w1483) -> (w1482:string)
                n1795 = Equal?(x=w1477, y=w1482) -> (x = y?=w1472:bool)
                n1796 = Concatenate Strings(w1473) -> (w1474:string)
                n1797 = Equal?(x=w1477, y=w1474) -> (x = y?=w1478:bool)
                n1798 = Or(x=w1472, y=w1478) -> (x .or. y?=w1471:bool)
                "x = y?" <- w1471
                n1799 = case shown="True" w1471 {
                  selector: w1471 -> [w1488 _]
                  tunnel: w1480 -> [_ _]
                  frame False {
                    n1800 = And(x=w1488, y=TRUE ("Visible")) -> (x .and. y?=w1489:bool)
                    n1801 = property on="message" class="Str"("Visible"=w1489) -> ()  [unwired: 2 in, 2 out]
                  }
                  frame True {
                    n1802 = property on="message" class="Str"("Visible"=FALSE) -> ()  [unwired: 2 in, 2 out]
                  }
                }
                n1803 = flat-sequence {
                  tunnel: [w1486] -> w1480
                  frame #0 {
                    w1486 = ""
                    n1804 = local write "Password"(w1486) -> ()
                  }
                }
              }
            }
          }
        }
        n1805 = case shown="True" "SrvM CP 2" {
          frame False {
          }
          frame True {
            n1806 = local read "FRIC. FORCE : 2"() -> (w1374:dbl)
            n1807 = local read "STROKE GAIN : 2"() -> (w1373:dbl)
            n1808 = local read "TEMPERATURE : 2"() -> (w1371:dbl)
            n1809 = local read "HUMIDITY: 2"() -> (w1369:dbl)
            n1810 = local read "DISPLACEMENT : 4"() -> (w1372:dbl)
            n1811 = local read "AIR TEMPERATURE : 2"() -> (w1370:dbl)
            n1812 = local read "TEMP INTERCEPT: 2"() -> (w1368:dbl)
            n1813 = local read "AIR TEMP INTERCEPT: 2"() -> (w1367:dbl)
            n1814 = local write "FRIC. FORCE :"(w1374) -> ()
            n1815 = local write "STROKE GAIN :"(w1373) -> ()
            n1816 = local write "TEMPERATURE :"(w1371) -> ()
            n1817 = local write "AIR TEMPERATURE :"(w1370) -> ()
            n1818 = local write "HUMIDITY:"(w1369) -> ()
            n1819 = local write "DISPLACEMENT :"(w1372) -> ()
            n1820 = local write "AIR TEMP INTERCEPT:"(w1368) -> ()
            n1821 = local write "TEMP INTERCEPT:"(w1367) -> ()
            n1822 = local write "SrvM CP 2"(FALSE ("SrvM CP 2")) -> ()
          }
        }
        n1823 = local read "STROKE GAIN : 2"() -> (w1343:dbl)
        n1824 = local read "FRIC. FORCE : 2"() -> (w1346:dbl)
        n1825 = local read "AIR TEMPERATURE : 2"() -> (w1334:dbl)
        n1826 = local read "DISPLACEMENT : 4"() -> (w1339:dbl)
        n1827 = local read "TEMPERATURE : 2"() -> (w1337:dbl)
        n1828 = local read "STROKE GAIN :"() -> (w1342:dbl)
        n1829 = local read "HUMIDITY: 2"() -> (w1330:dbl)
        n1830 = local read "FRIC. FORCE :"() -> (w1345:dbl)
        n1831 = local read "AIR TEMPERATURE :"() -> (w1333:dbl)
        n1832 = local read "DISPLACEMENT :"() -> (w1338:dbl)
        n1833 = local read "TEMPERATURE :"() -> (w1335:dbl)
        n1834 = local read "HUMIDITY:"() -> (w1329:dbl)
        n1835 = Subtract(x=w1330, y=w1329) -> (x-y=w1331:dbl)
        n1836 = Subtract(x=w1343, y=w1342) -> (x-y=w1341:dbl)
        n1837 = Subtract(x=w1346, y=w1345) -> (x-y=w1344:dbl)
        n1838 = Subtract(x=w1337, y=w1335) -> (x-y=w1336:dbl)
        n1839 = Subtract(x=w1339, y=w1338) -> (x-y=w1340:dbl)
        n1840 = Subtract(x=w1334, y=w1333) -> (x-y=w1332:dbl)
        n1841 = Divide(x=w1341, y=w1342) -> (x/y=w1361:dbl)
        n1842 = Divide(x=w1332, y=w1333) -> (x/y=w1356:dbl)
        n1843 = Divide(x=w1344, y=w1345) -> (x/y=w1364:dbl)
        n1844 = Divide(x=w1331, y=w1329) -> (x/y=w1353:dbl)
        n1845 = Divide(x=w1336, y=w1335) -> (x/y=w1357:dbl)
        n1846 = Divide(x=w1340, y=w1338) -> (x/y=w1360:dbl)
        n1847 = Multiply(x=w1361, y=100.0) -> (x*y=→"STROKE Calibration Error":dbl)
        n1848 = Multiply(x=w1356, y=100.0) -> (x*y=→"AIR TEMPERATURE  Calibration Error":dbl)
        n1849 = Multiply(x=w1364, y=100.0) -> (x*y=→"FRIC. FORCE Calibration Error":dbl)
        n1850 = Multiply(x=w1360, y=100.0) -> (x*y=→"DISPLACEMENT  Calibration Error":dbl)
        n1851 = Multiply(x=w1353, y=100.0) -> (x*y=→"HUMIDITY  Calibration Error":dbl)
        n1852 = Multiply(x=w1357, y=100.0) -> (x*y=→"TEMPERATURE  Calibration Error":dbl)
      }
    }
  }
  n1853 = while {
    tunnel: [w2816] -> _
    tunnel: [w2815] -> w38
    tunnel: w15 -> [_]
    i -> [w2816]
    stop <- w2815 stop-if-true
    n1854 = local read "Main Tab"() -> (w2801:T2)
    n1855 = local read "EDIT"() -> (w2822:bool)
    n1856 = case shown="True" w2822 {
      tunnel: [FALSE TRUE] -> w2807
      frame False {
      }
      frame True {
      }
    }
    n1857 = local read "Rate"() -> (w2821:dbl)
    n1858 = Divide(x=1.0, y=w2821) -> (x/y=w2817:dbl)
    "Time 2" <- w2817
    n1859 = property on="Time slide" class="Slide (strict)"("Scale.Range:Maximum"=2500.0) -> ()  [unwired: 2 in, 2 out]
    n1860 = local read "conststatus"() -> (w2803:dbl)
    n1861 = Equal?(x=w2801, y=T15."About" ("Main Tab")) -> (x = y?=w2813:bool)
    n1862 = property on="FF Calibration g" class="WFGraph (strict)"("Visible"=w2807) -> ()  [unwired: 2 in, 2 out]
    n1863 = property on="Lift" class="Bool (strict)"("Visible"=w2807) -> ()  [unwired: 2 in, 2 out]
    n1864 = property on="Threshold" class="DigNum (strict)"("Visible"=w2807) -> ()  [unwired: 2 in, 2 out]
    n1865 = property on="Time slide" class="Slide (strict)"("Visible"=w2807) -> ()  [unwired: 2 in, 2 out]
    n1866 = Select(t=u32 2500 ("milliseconds to wait"), s=w2813, f=u32 500 ("milliseconds to wait")) -> (s? t:f=w2811:u32)
    n1867 = Multiply(x=w2817, y=w2811) -> (x*y=w2819:dbl)
    n1868 = Wait (ms)(milliseconds to wait=u32 50) -> ()  [unwired: 1 out]
    n1869 = call "Elapsed Time2"("Time Target (s)"=w2819, "Auto Reset"=TRUE) -> ("Time has Elapsed"=w2808:bool)  [unwired: 10 in, 7 out]
    n1870 = Equal?(x=w2803, y=0.0) -> (x = y?=w2804:bool)
    n1871 = case shown="True" w2804 {
      frame False {
      }
      frame True {
        # "C:\\WinDucom\\calibrate WO 2391.dcf"
        n1872 = local write "Lan flag"(22) -> ()
        n1873 = local write "conststatus"(10.0 ("rpm value : 2")) -> ()
        n1874 = String To Path(string="C:\\LAB-IQ-NXT\\calibrate WO 2464.dcf") -> (path=w2828:path)
        n1875 = Open/Create/Replace File "Open File"(file path (use dialog)=w2828) -> (refnum out=w2826:refnum<file>)  [unwired: 5 in, 2 out]
        n1876 = for {
          N: 22 -> [_]
          tunnel: w2826 -> [w2837]
          i -> [w2831]
          (unwired) TRUE ("line mode (F)")
          n1877 = Read from Text File "Read File"(file (use dialog)=w2837) -> (text=w2836:string)  [unwired: 3 in, 3 out]
          n1878 = Match Pattern(string=w2836, regular expression="]") -> (after substring=w2834:string)  [unwired: 1 in, 3 out]
          n1879 = String Subset(string=w2836, offset (0)=5, length (rest)=10 ("length (rest)")) -> (substring=w2829:string)
          n1880 = Fract/Exp String To Number(string=w2829) -> (number=w2830:dbl)  [unwired: 3 in, 1 out]
          n1881 = Match Pattern(string=w2834, regular expression="-") -> (before substring=w2832:string)  [unwired: 1 in, 3 out]
          n1882 = case shown="11" w2831 {
            tunnel: w2830 -> [w2840 w2841 w2842 w2843 _ _ _ w2848 w2849 w2850 w2853 w2854 w2855 w2856 w2857 w2858 w2859 w2862 w2863 _ _ w2866 _]
            tunnel: w2832 -> [_ _ _ _ w2844 w2845 w2846 _ _ _ _ _ _ _ _ _ _ _ _ w2864 w2865 _ _]
            frame 0 {
              n1883 = local write "FRIC. FORCE :"(w2840) -> ()
            }
            frame 1 {
              n1884 = local write "TEMPERATURE :"(w2841) -> ()
            }
            frame 2 {
              n1885 = local write "HUMIDITY:"(w2842) -> ()
            }
            frame 3 {
              n1886 = local write "AIR TEMPERATURE :"(w2843) -> ()
            }
            frame 4 {
